vi "labview_nanonisKernel.vi"(3 "Error in (no error)":errorcluster, 4 "Input":string, 5 "Application ref in":refnum<vi>) -> (0 "Error out":errorcluster, 2 "Output":string)   [LabVIEW 2019]
uses:
  <userlib>/Nanonis Prog Interface/Scan/Grid/GridPatternGet.vi
  <userlib>/Nanonis Prog Interface/Nanonis Prog Interface.lvlib
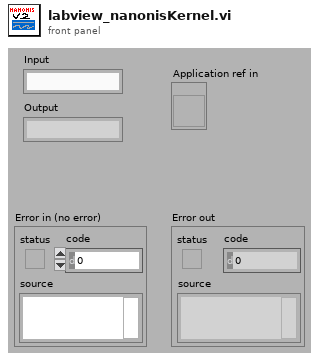
[diagram p1: front panel]
types:
  T1 = enum16{"no change", "home absolute", "home relative"}
  T2 = enum8{"Group 1", "Group 2", "Group 3", "Group 4", "Group 5", "Group 6"}
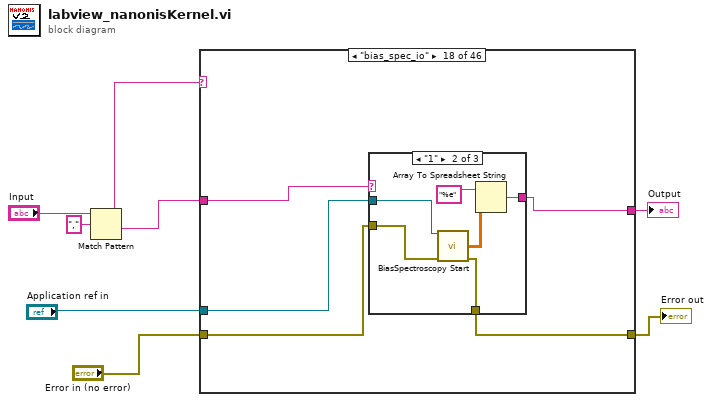
[diagram p0: block diagram]
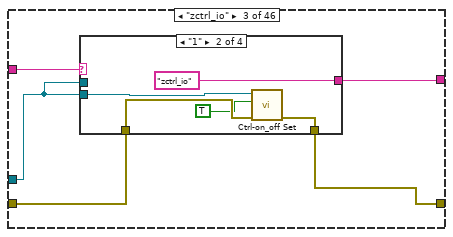
[diagram p4: hidden frame]
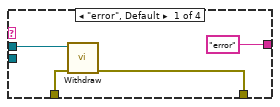
[diagram p5: hidden frame]
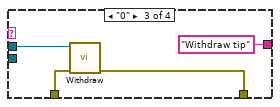
[diagram p6: hidden frame]
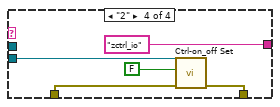
[diagram p7: hidden frame]
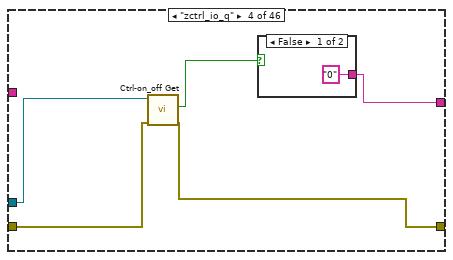
[diagram p8: hidden frame]
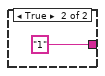
[diagram p9: hidden frame]
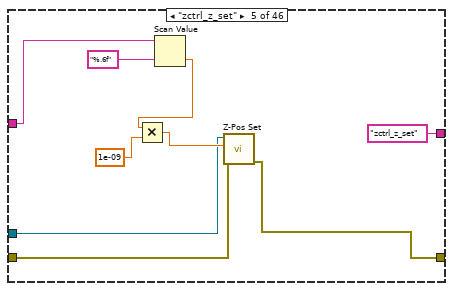
[diagram p10: hidden frame]
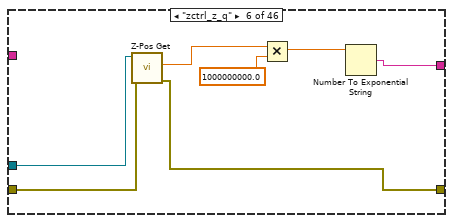
[diagram p11: hidden frame]
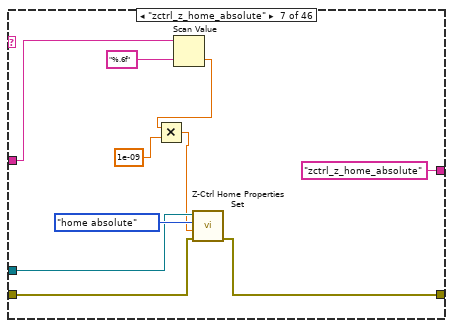
[diagram p12: hidden frame]
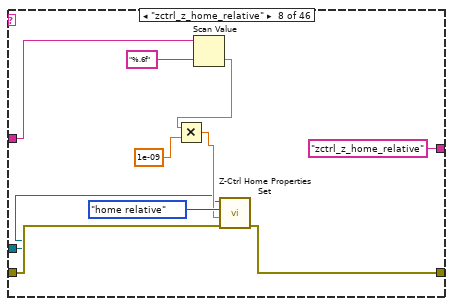
[diagram p13: hidden frame]
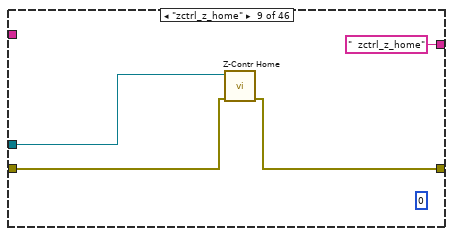
[diagram p14: hidden frame]
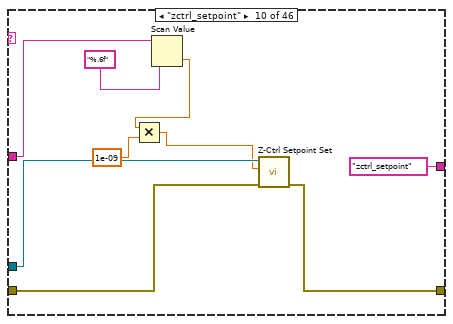
[diagram p15: hidden frame]
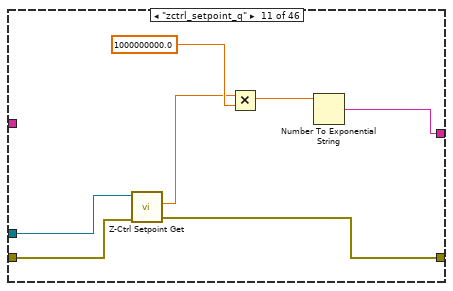
[diagram p16: hidden frame]
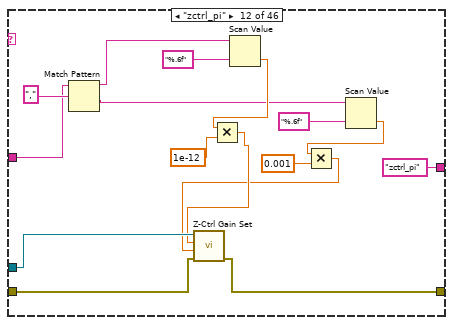
[diagram p17: hidden frame]
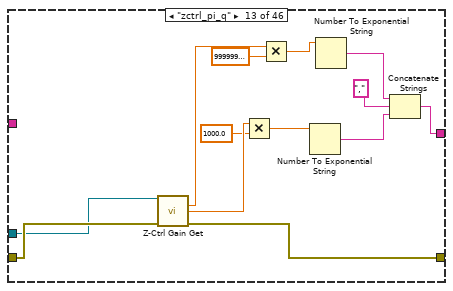
[diagram p18: hidden frame]
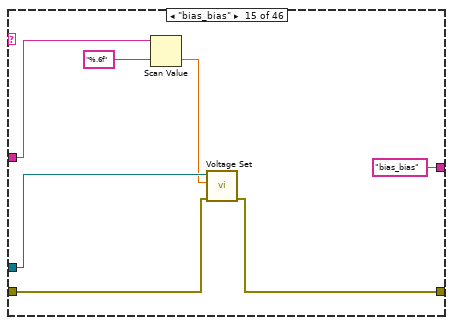
[diagram p20: hidden frame]
diagram:
  n1 = Match Pattern(string="Input", regular expression=",") -> (before substring=w5:string, after substring=w4:string)  [unwired: 1 in, 2 out]
  n2 = case shown="\"bias_spec_io\"" w5 {
    tunnel: [w10 w12 w16 w37 "zctrl_z_set" ("Input") w53 "zctrl_z_home_absolute" ("Input") "zctrl_z_home_relative" ("Input") "  zctrl_z_home" ("Input") "zctrl_setpoint" ("Input") w96 "zctrl_pi" ("Input") w115 w129 "bias_bias" ("Input") w138 "bias_pulse" ("Input") w163 w180 "bias_spec_sweep" ("Input") w199 "  bias_spec_channel" ("Input") w217 w219 w220 w223 w225 w227 w230 w255 w269 w295 w319 w330 w351 w360 w377 w389 w397 w412 w420 w436 "1" ("regular expression") w447 w461 w469] -> w8
    tunnel: w4 -> [w10 w12 w17 _ w50 _ w59 w69 _ w83 _ w106 _ w129 w130 _ w149 w162 _ w187 _ w213 w217 w219 w220 w223 w225 w227 w236 w256 w270 w297 w311 w342 w359 w365 w378 _ w408 _ _ w435 _ _ _ w469]
    tunnel: "Error in (no error)" -> [w9 w11 w15 w39 w45 w57 w66 w76 w82 w91 w94 w113 w127 w128 w136 w141 w156 w165 w178 w195 w204 w212 w216 w218 w221 w222 w224 w226 w235 w259 w272 w305 w326 w341 w355 w363 w376 w388 _ w418 w423 w432 w445 w451 w467 w478]
    tunnel: "Application ref in" -> [_ _ w14 w40 w46 w58 w64 w70 w79 w90 w95 w112 w125 _ w133 w140 w155 w161 w177 w193 w196 w210 _ _ _ _ _ _ w234 w260 w271 w306 w327 w340 w356 w364 w375 w386 w400 w419 w424 w431 w443 w450 w468 w476]
    tunnel: [w9 w11 w13 w36 w43 w52 w65 w75 w81 w89 w93 w111 w126 w128 w135 w139 w154 w164 w179 w194 w203 w211 w216 w218 w221 w222 w224 w226 w233 w246 w268 w302 w325 w335 w354 w361 w372 w387 w399 w417 w421 w430 w444 w449 w466 w477] -> w2
    frame "test", Default {
    }
    frame "###z controller###" {
    }
    frame "zctrl_io" {
      n3 = case shown="\"1\"" w17 {
        tunnel: ["error" ("regular expression") "zctrl_io" ("regular expression") "Withdraw tip" ("regular expression") "zctrl_io" ("regular expression")] -> w16
        tunnel: w14 -> [w19 _ w30 _]
        tunnel: w15 -> [w20 w25 w29 w31]
        tunnel: w14 -> [_ w23 _ w33]
        tunnel: [w18 w22 w27 w34] -> w13
        frame "error", Default {
          n4 = call <userlib>:"Withdraw.vi"("Error in (no error)"=w20, "Application ref in"=w19) -> ("Error out"=w18:errorcluster)  [unwired: 8 in, 1 out]
        }
        frame "1" {
          n5 = call <userlib>:"Ctrl-on_off Set.vi"("error in (no error)"=w25, "Z Controller ON/OFF"=TRUE ("Lockin ON/OFF"), "Application ref in"=w23) -> ("error out"=w22:errorcluster)  [unwired: 7 in, 1 out]
        }
        frame "0" {
          n6 = call <userlib>:"Withdraw.vi"("Error in (no error)"=w29, "Application ref in"=w30) -> ("Error out"=w27:errorcluster)  [unwired: 8 in, 1 out]
        }
        frame "2" {
          n7 = call <userlib>:"Ctrl-on_off Set.vi"("error in (no error)"=w31, "Z Controller ON/OFF"=FALSE ("Lockin ON/OFF"), "Application ref in"=w33) -> ("error out"=w34:errorcluster)  [unwired: 7 in, 1 out]
        }
      }
    }
    frame "zctrl_io_q" {
      n8 = call <userlib>:"Ctrl-on_off Get.vi"("error in (no error)"=w39, "Application ref in"=w40) -> ("error out"=w36:errorcluster, "Z-Controller on/off status"=w38:bool)  [unwired: 7 in, 1 out]
      n9 = case shown="False" w38 {
        tunnel: ["0" "1"] -> w37
        frame False {
        }
        frame True {
        }
      }
    }
    frame "zctrl_z_set" {
      n10 = Scan Value(string=w50, format string="%.6f") -> (value=w48:dbl)  [unwired: 1 in, 1 out]
      n11 = Multiply(x=w48, y=1e-09) -> (x*y=w47:dbl)
      n12 = call <userlib>:"Z-Pos Set.vi"("error in (no error)"=w45, "Z position (m)"=w47, "Application ref in"=w46) -> ("error out"=w43:errorcluster)  [unwired: 7 in, 1 out]
    }
    frame "zctrl_z_q" {
      n13 = call <userlib>:"Z-Pos Get.vi"("error in (no error)"=w57, "Application ref in"=w58) -> ("error out"=w52:errorcluster, "Z position (m)"=w55:sgl)  [unwired: 7 in, 1 out]
      n14 = Multiply(x=w55, y=1000000000.0) -> (x*y=w54:dbl)
      n15 = Number To Exponential String(number=w54) -> (E-format string=w53:string)  [unwired: 3 in]
    }
    frame "zctrl_z_home_absolute" {
      n16 = Scan Value(string=w59, format string="%.6f") -> (value=w61:dbl)  [unwired: 1 in, 1 out]
      n17 = Multiply(x=w61, y=1e-09) -> (x*y=w60:dbl)
      n18 = call <userlib>:"Z-Ctrl Home Properties Set.vi"("error in (no error)"=w66, "Home position (m) (NaN=no change)"=w60, "Absolute/Relative Switch (no change=Default)"=T1."home absolute", "Application ref in"=w64) -> ("error out"=w65:errorcluster)  [unwired: 5 in, 1 out]
    }
    frame "zctrl_z_home_relative" {
      n19 = Scan Value(string=w69, format string="%.6f") -> (value=w72:dbl)  [unwired: 1 in, 1 out]
      n20 = Multiply(x=w72, y=1e-09) -> (x*y=w71:dbl)
      n21 = call <userlib>:"Z-Ctrl Home Properties Set.vi"("error in (no error)"=w76, "Home position (m) (NaN=no change)"=w71, "Absolute/Relative Switch (no change=Default)"=T1."home relative", "Application ref in"=w70) -> ("error out"=w75:errorcluster)  [unwired: 5 in, 1 out]
    }
    frame "zctrl_z_home" {
      (unwired) 0
      n22 = call <userlib>:"Z-Contr Home.vi"("Error in (no error)"=w82, "Application ref in"=w79) -> ("Error out"=w81:errorcluster)  [unwired: 8 in, 1 out]
    }
    frame "zctrl_setpoint" {
      n23 = Scan Value(string=w83, format string="%.6f") -> (value=w86:dbl)  [unwired: 1 in, 1 out]
      n24 = Multiply(x=w86, y=1e-09) -> (x*y=w85:dbl)
      n25 = call <userlib>:"Z-Ctrl Setpoint Set.vi"("error in (no error)"=w91, "Z Controller setpoint"=w85, "Application ref in"=w90) -> ("error out"=w89:errorcluster)  [unwired: 7 in, 1 out]
    }
    frame "zctrl_setpoint_q" {
      n26 = call <userlib>:"Z-Ctrl Setpoint Get.vi"("error in (no error)"=w94, "Application ref in"=w95) -> ("error out"=w93:errorcluster, "Z Controller setpoint"=w92:sgl)  [unwired: 6 in, 1 out]
      n27 = Multiply(x=w92, y=1000000000.0) -> (x*y=w97:dbl)
      n28 = Number To Exponential String(number=w97) -> (E-format string=w96:string)  [unwired: 3 in]
    }
    frame "zctrl_pi" {
      n29 = Match Pattern(string=w106, regular expression=",") -> (before substring=w105:string, after substring=w102:string)  [unwired: 1 in, 2 out]
      n30 = Scan Value(string=w105, format string="%.6f") -> (value=w108:dbl)  [unwired: 1 in, 1 out]
      n31 = Multiply(x=w108, y=1e-12) -> (x*y=w104:dbl)
      n32 = Scan Value(string=w102, format string="%.6f") -> (value=w101:dbl)  [unwired: 1 in, 1 out]
      n33 = Multiply(x=w101, y=0.001) -> (x*y=w100:dbl)
      n34 = call <userlib>:"Z-Ctrl Gain Set.vi"("error in (no error)"=w113, "Time constant (s)"=w100, "P-gain"=w104, "Application ref in"=w112) -> ("error out"=w111:errorcluster)  [unwired: 5 in, 1 out]
    }
    frame "zctrl_pi_q" {
      n35 = call <userlib>:"Z-Ctrl Gain Get.vi"("Application ref in"=w125, "error in (no error)"=w127) -> ("P-gain"=w122:sgl, "Time constant (s)"=w121:sgl, "error out"=w126:errorcluster)  [unwired: 9 in, 2 out]
      n36 = Multiply(x=w121, y=sgl 1000.0) -> (x*y=w123:sgl)
      n37 = Multiply(x=w122, y=sgl 1000000000000.0) -> (x*y=w124:sgl)
      n38 = Number To Exponential String(number=w123) -> (E-format string=w116:string)  [unwired: 3 in]
      n39 = Number To Exponential String(number=w124) -> (E-format string=w117:string)  [unwired: 3 in]
      n40 = Concatenate Strings(w117, "," ("string"), w116) -> (w115:string)
    }
    frame "###Bias/Bias Spectrum###" {
    }
    frame "bias_bias" {
      n41 = Scan Value(string=w130, format string="%.6f") -> (value=w132:dbl)  [unwired: 1 in, 1 out]
      n42 = call <userlib>:"Voltage Set.vi"("Error in (no error)"=w136, "Bias (V)"=w132, "Application ref in"=w133) -> ("Error out"=w135:errorcluster)  [unwired: 7 in, 1 out]
    }
    frame "bias_bias_q" {
      n43 = call <userlib>:"Voltage Get.vi"("error in (no error)"=w141, "Application ref in"=w140) -> ("error out"=w139:errorcluster, "Bias (V)"=w137:sgl)  [unwired: 7 in, 1 out]
      n44 = Number To Exponential String(number=w137) -> (E-format string=w138:string)  [unwired: 3 in]
    }
    frame "bias_pulse" {
      w146 = "," ("regular expression")
      n45 = Match Pattern(string=w149, regular expression=w146) -> (before substring=w151:string, after substring=w144:string)  [unwired: 1 in, 2 out]
      n46 = Match Pattern(string=w144, regular expression=w146) -> (before substring=w145:string, after substring=w143:string)  [unwired: 1 in, 2 out]
      n47 = Scan Value(string=w151, format string="%.6f") -> (value=w148:dbl)  [unwired: 1 in, 1 out]
      n48 = case shown="\"0\"" w143 {
        tunnel: [enum16{"no change", "hold", "don't hold"}."no change" ("Z-Controller (no change)") enum16{"no change", "hold", "don't hold"}."hold" ("Z-Controller (no change)") enum16{"no change", "hold", "don't hold"}."don't hold" ("Z-Controller (no change)")] -> w142
        frame Default {
        }
        frame "1" {
        }
        frame "0" {
        }
      }
      n49 = Scan Value(string=w145, format string="%.6f") -> (value=w147:dbl)  [unwired: 1 in, 1 out]
      n50 = call <userlib>:"Bias Pulse.vi"("Application ref in"=w155, "Pulse bias (V) (1)"=w148, "Pulse width (s) (100m)"=w147, "Z-Controller (no change)"=w142, "Error in (no error)"=w156, "Pulse abs/rel (no change)"=enum16{"no change", "relative", "absolute"}."absolute") -> ("Error out"=w154:errorcluster)  [unwired: 8 in, 1 out]
    }
    frame "bias_spec_io" {
      n51 = case shown="\"1\"" w162 {
        tunnel: ["Error!" ("regular expression") w169 "STS stop" ("regular expression")] -> w163
        tunnel: w165 -> [w166 w172 w175]
        tunnel: w161 -> [_ w173 _]
        tunnel: [w166 w171 w174] -> w164
        frame "error", Default {
        }
        frame "1" {
          n52 = call <userlib>:"BiasSpectroscopy Start.vi"("Application ref in"=w173, "Error in (no error)"=w172) -> ("Data"=w168:sgl[][], "Error out"=w171:errorcluster)  [unwired: 9 in, 3 out]
          n53 = Array To Spreadsheet String(array=w168, 3:"%e" ("format string")) -> (spreadsheet string=w169:string)  [unwired: 1 in]
        }
        frame "0" {
          n54 = call <userlib>:"BiasSpectroscopy Stop.vi"("Error in (no error)"=w175) -> ("Error out"=w174:errorcluster)  [unwired: 13 in, 1 out]
        }
      }
    }
    frame "bias_spec_q" {
      n55 = call <userlib>:"BiasSpectroscopy Status Get.vi"("Error in (no error)"=w178, "Application ref in"=w177) -> ("Error out"=w179:errorcluster, "Running?"=w181:bool)  [unwired: 5 in, 1 out]
      n56 = case shown="True" w181 {
        tunnel: ["0" "1"] -> w180
        frame False {
        }
        frame True {
        }
      }
    }
    frame "bias_spec_sweep" {
      n57 = Match Pattern(string=w187, regular expression=",") -> (before substring=w190:string, after substring=w188:string)  [unwired: 1 in, 2 out]
      n58 = Scan Value(string=w190, format string="%.6f") -> (value=w186:dbl)  [unwired: 1 in, 1 out]
      n59 = Scan Value(string=w188, format string="%.6f") -> (value=w185:dbl)  [unwired: 1 in, 1 out]
      n60 = call <userlib>:"BiasSpectroscopy SetLimits.vi"("Error in (no error)"=w195, "End value (V)"=w185, "Start value (V)"=w186, "Application ref in"=w193) -> ("Error out"=w194:errorcluster)  [unwired: 4 in, 1 out]
    }
    frame "bias_spec_sweep_q" {
      n61 = call <userlib>:"BiasSpectroscopy GetLimits.vi"("Error in (no error)"=w204, "Application ref in"=w196) -> ("Error out"=w203:errorcluster, "End value (V)"=w198:sgl, "Start value (V)"=w197:sgl)  [unwired: 4 in, 1 out]
      n62 = Number To Exponential String(number=w198) -> (E-format string=w200:string)  [unwired: 3 in]
      n63 = Number To Exponential String(number=w197) -> (E-format string=w201:string)  [unwired: 3 in]
      n64 = Concatenate Strings(w201, "," ("string"), w200) -> (w199:string)
    }
    frame "bias_spec_channel" {
      n65 = Spreadsheet String To Array(delimiter (Tab)=",", format string="", spreadsheet string=w213) -> (array=w208:dbl[][])  [unwired: 1 in]
      n66 = Array Size(array=w208) -> (size(s)=w209:i32[])
      n67 = Array Max & Min(array=w209) -> (max value=w207:i32)  [unwired: 3 out]
      n68 = Reshape Array(w208, w207) -> (w206:dbl[])
      n69 = call <userlib>:"BiasSpectroscopy Channels Set.vi"("Error in (no error)"=w212, "Channels"=w206, "Application ref in"=w210) -> ("Error out"=w211:errorcluster)  [unwired: 7 in, 1 out]
    }
    frame "###Current###" {
    }
    frame "###Walker###" {
    }
    frame "###Move/Drift/Tilt###" {
    }
    frame "###Scan###" {
    }
    frame "###Grid###" {
    }
    frame "###LockIn###" {
    }
    frame "WLK_S" {
      w239 = "," ("regular expression")
      # "Frequency"
      # "Voltage"
      n70 = Match Pattern(string=w236, regular expression=w239) -> (before substring=w232:string, after substring=w240:string)  [unwired: 1 in, 2 out]
      n71 = Match Pattern(string=w240, regular expression=w239) -> (before substring=w231:string)  [unwired: 1 in, 3 out]
      n72 = Decimal String To Number(string=w231) -> (number=w238:i32)  [unwired: 2 in, 1 out]
      n73 = Decimal String To Number(string=w232) -> (number=w237:i32)  [unwired: 2 in, 1 out]
      n74 = call <userlib>:"Motor Frequency Amplitude Set.vi"("Error in (no error)"=w235, "Amplitude (V) (NaN=no change)"=w237, "Frequency (Hz) (NaN=no change)"=w238, "Application ref in"=w234) -> ("Error out"=w233:errorcluster)  [unwired: 6 in, 1 out]
      n75 = Concatenate Strings("WLK_S, V:  " ("string"), w232, ", F: " ("string"), w231) -> (w230:string)
    }
    frame "WLK_W" {
      w252 = "," ("string")
      # "Steps"
      # "Direction"
      n76 = Match Pattern(string=w256, regular expression=w252) -> (before substring=w242:string, after substring=w258:string)  [unwired: 1 in, 2 out]
      n77 = case shown="\"False\", Default" w242 {
        tunnel: [-1 0 1 2 3 4 5] -> w241
        frame "False", Default {
        }
        frame "+X", "+x", "0", "X+", "x+" {
        }
        frame "-X", "-x", "1", "X-", "x-" {
        }
        frame "+Y", "+y", "2", "Y+", "y+" {
        }
        frame "-Y", "-y", "3", "Y-", "y-" {
        }
        frame "+Z", "+z", "4", "Z+", "z+" {
        }
        frame "-Z", "-z", "5", "Z-", "z-" {
        }
      }
      n78 = Match Pattern(string=w258, regular expression=w252) -> (before substring=w257:string)  [unwired: 1 in, 3 out]
      n79 = Decimal String To Number(string=w257) -> (number=w250:i32)  [unwired: 2 in, 1 out]
      n80 = call <userlib>:"Motor Start Move.vi"("Group"=T2."Group 4", "Error in (no error)"=w259, "Number of steps"=w250, "Direction"=w241, "Application ref in"=w260) -> ("Error out"=w245:errorcluster, "Application ref out"=w251:refnum<vi>)  [unwired: 4 in]
      n81 = Concatenate Strings("WLK_W, Dir: " ("string"), w242, ", Steps: " ("string"), w257) -> (w255:string)
      n82 = call <userlib>:"Motor Frequency Amplitude Get.vi"("Application ref in"=w251) -> ("Frequency (Hz)"=w249:sgl)  [unwired: 7 in, 3 out]
      n83 = Divide(x=w250, y=w249) -> (x/y=w248:sgl)
      n84 = Add(x=w248, y=sgl 0.5) -> (x+y=w244:sgl)
      n85 = call "Time Delay"("error in (no error)"=w245, "Delay Time (s)"=w244) -> ("error out"=w246:errorcluster)  [unwired: 9 in]
    }
    frame "WLK_W5" {
      w281 = "," ("string")
      # "Steps"
      # "Direction"
      n86 = Match Pattern(string=w270, regular expression=w281) -> (before substring=w286:string, after substring=w287:string)  [unwired: 1 in, 2 out]
      n87 = Match Pattern(string=w287, regular expression=w281) -> (before substring=w285:string)  [unwired: 1 in, 3 out]
      n88 = Decimal String To Number(string=w285) -> (number=w279:i32)  [unwired: 2 in, 1 out]
      n89 = Decimal String To Number(string=w286) -> (number=w284:i32)  [unwired: 2 in, 1 out]
      n90 = Concatenate Strings("WLK_W, Dir: " ("string"), w286, ", Steps: " ("string"), w285) -> (w269:string)
      n91 = call <userlib>:"Motor Start Move.vi"("Group"=T2."Group 5", "Error in (no error)"=w272, "Number of steps"=w279, "Direction"=w284, "Application ref in"=w271) -> ("Error out"=w275:errorcluster, "Application ref out"=w280:refnum<vi>)  [unwired: 4 in]
      n92 = call <userlib>:"Motor Frequency Amplitude Get.vi"("Application ref in"=w280) -> ("Frequency (Hz)"=w278:sgl)  [unwired: 7 in, 3 out]
      n93 = Divide(x=w279, y=w278) -> (x/y=w277:sgl)
      n94 = Add(x=w277, y=sgl 0.5) -> (x+y=w274:sgl)
      n95 = call "Time Delay2"("error in (no error)"=w275, "Delay Time (s)"=w274) -> ("error out"=w268:errorcluster)  [unwired: 9 in]
    }
    frame "RD_I" {
      w300 = "," ("regular expression")
      # "AVG#"
      # "Index"
      n96 = Match Pattern(string=w297, regular expression=w300) -> (before substring=w299:string, after substring=w301:string)  [unwired: 1 in, 2 out]
      n97 = Match Pattern(string=w301, regular expression=w300) -> (before substring=w298:string)  [unwired: 1 in, 3 out]
      n98 = call <userlib>:"Signal Names Get.vi"("error in (no error)"=w305, "Application ref in"=w306) -> ("error out"=w304:errorcluster, "Signals Names"=w294:string[], "Application ref out"=w303:refnum<vi>)  [unwired: 5 in]
      n99 = Decimal String To Number(string=w298) -> (number=w296:i32)  [unwired: 2 in, 1 out]
      n100 = Decimal String To Number(string=w299) -> (number=w293:i32)  [unwired: 2 in, 1 out]
      n101 = Index Array(array=w294, index=w293) -> (element=w291:string)
      n102 = call "Nanonis_read IO.vi"("error in (no error)"=w304, "Num Average"=w296, "Signal index (0-23)"=w293, "Application ref in"=w303) -> ("error out"=w302:errorcluster, "DC value"=w289:ext)
      n103 = Format Value(format string="%e", value (0)=w289) -> (output string=w290:string)  [unwired: 1 in]
      n104 = Concatenate Strings(w291, "," ("string"), w290) -> (w295:string)
    }
    frame "APP" {
      w307 = "," ("regular expression")
      # "100ms"
      n105 = Match Pattern(string=w311, regular expression=w307) -> (before substring=w317:string, after substring=w318:string)  [unwired: 1 in, 2 out]
      n106 = Match Pattern(string=w318, regular expression=w307) -> (before substring=w316:string, after substring=w308:string)  [unwired: 1 in, 2 out]
      n107 = Match Pattern(string=w308, regular expression=w307) -> (before substring=w309:string)  [unwired: 1 in, 3 out]
      n108 = Decimal String To Number(string=w309) -> (number=w310:i32)  [unwired: 2 in, 1 out]
      n109 = Decimal String To Number(string=w316) -> (number=w314:i32)  [unwired: 2 in, 1 out]
      n110 = Multiply(x=w314, y=1000) -> (x*y=w312:i32)
      n111 = Decimal String To Number(string=w317) -> (number=w315:i32)  [unwired: 2 in, 1 out]
      n112 = call "Nanonis_autoAPP.vi"("Application reference"=w327, "steps"=w315, "Number of pulses"=w310, "Wait for motor (ms)"=w312, "Error in (no error)"=w326) -> ("Surface reached"=w324:bool, "Total steps"=w320:u32, "error out"=w325:errorcluster)  [unwired: 1 in]
      n113 = case shown="False" w324 {
        tunnel: ["0" ("regular expression") "1" ("regular expression")] -> w323
        frame False {
        }
        frame True {
        }
      }
      n114 = Number To Decimal String(number=w320) -> (decimal integer string=w321:string)  [unwired: 1 in]
      n115 = Concatenate Strings(w323, "," ("string"), w321) -> (w319:string)
    }
    frame "LCK_S" {
      w336 = "%.6f" ("format string")
      w343 = "," ("string")
      w332 = "," ("string")
      # "Frequency"
      # "Phase"
      # "Amplitude"
      n116 = Match Pattern(string=w342, regular expression=w343) -> (before substring=w334:string, after substring=w344:string)  [unwired: 1 in, 2 out]
      n117 = Match Pattern(string=w344, regular expression=w343) -> (before substring=w333:string, after substring=w345:string)  [unwired: 1 in, 2 out]
      n118 = Match Pattern(string=w345, regular expression=w343) -> (before substring=w331:string)  [unwired: 1 in, 3 out]
      n119 = Scan Value(string=w331, format string=w336) -> (value=w337:dbl)  [unwired: 1 in, 1 out]
      n120 = Decimal String To Number(string=w334) -> (number=w339:i32)  [unwired: 2 in, 1 out]
      n121 = Scan Value(string=w333, format string=w336) -> (value=w338:dbl)  [unwired: 1 in, 1 out]
      n122 = call <userlib>:"Lockin Modulation param Set.vi"("Application ref in"=w340, "Amplitude (mod. signal unit) (NaN = no change)"=w338, "Frequency (Hz) (NaN = no change)"=w339, "Ref Phase (deg) (NaN = no change)"=w337, "Error in (no error)"=w341) -> ("Error out"=w335:errorcluster)  [unwired: 9 in, 1 out]
      n123 = Concatenate Strings(w334, w332, w333, w332, w331) -> (w330:string)
    }
    frame "LCK_M" {
      w358 = "," ("regular expression")
      # "Demod"
      # "Mod"
      n124 = Match Pattern(string=w359, regular expression=w358) -> (before substring=w349:string, after substring=w357:string)  [unwired: 1 in, 2 out]
      n125 = Match Pattern(string=w357, regular expression=w358) -> (before substring=w346:string)  [unwired: 1 in, 3 out]
      n126 = Decimal String To Number(string=w349) -> (number=w353:i32)  [unwired: 2 in, 1 out]
      n127 = Decimal String To Number(string=w346) -> (number=w352:i32)  [unwired: 2 in, 1 out]
      n128 = call <userlib>:"Lockin MoDem Signal Set.vi"("Error in (no error)"=w355, "Demod. index"=w352, "Mod. index"=w353, "Application ref in"=w356) -> ("Error out"=w354:errorcluster)  [unwired: 6 in, 1 out]
      n129 = Concatenate Strings("Mod: " ("string"), w349, "," ("string"), "Demod" ("string"), w346) -> (w351:string)
    }
    frame "LCK_IO" {
      n130 = case shown="\"0\"" w365 {
        tunnel: [FALSE ("Lockin ON/OFF") TRUE ("Lockin ON/OFF") FALSE ("Lockin ON/OFF")] -> w362
        tunnel: ["Error!" ("regular expression") "Lockin on" ("regular expression") "Lockin off" ("regular expression")] -> w360
        frame "error", Default {
        }
        frame "1" {
        }
        frame "0" {
        }
      }
      n131 = call <userlib>:"Lockin on_off Set.vi"("Error in (no error)"=w363, "Lockin ON/OFF"=w362, "Application ref in"=w364) -> ("Error out"=w361:errorcluster)  [unwired: 7 in, 1 out]
    }
    frame "SCAN_IO" {
      (unwired) 0
      n132 = case shown="\"start\"" w378 {
        tunnel: ["Error!" ("regular expression") "Scan start" ("regular expression") "Scan stop" ("regular expression")] -> w377
        tunnel: [enum16{"Start", "Stop", "Pause", "Resume"}."Pause" ("Scan action (Start)") enum16{"Start", "Stop", "Pause", "Resume"}."Start" ("Scan action (Start)") enum16{"Start", "Stop", "Pause", "Resume"}."Stop" ("Scan action (Start)")] -> w374
        frame "error", Default {
        }
        frame "start" {
        }
        frame "stop" {
          (unwired) FALSE ("Lockin ON/OFF")
        }
      }
      n133 = call <userlib>:"Scan Action.vi"("error in (no error)"=w376, "Direction: up/down (T=up)"=TRUE, "Scan action (Start)"=w374, "Application ref in"=w375) -> ("error out"=w372:errorcluster)  [unwired: 5 in, 1 out]
    }
    frame "SCAN_STAT" {
      (unwired) 0
      n134 = call <userlib>:"Scan Status Get.vi"("error in (no error)"=w388, "Application ref in"=w386) -> ("error out"=w387:errorcluster, "Scanning?"=w385:bool)  [unwired: 6 in, 1 out]
      n135 = case shown="False" w385 {
        tunnel: ["0" "1"] -> w389
        frame False {
        }
        frame True {
        }
      }
    }
    frame "SCAN_FRAME" {
      (unwired) 0
      w403 = "," ("regular expression")
      # "size"
      # "Y"
      # "X"
      n136 = Match Pattern(string=w408, regular expression=w403) -> (before substring=w396:string, after substring=w409:string)  [unwired: 1 in, 2 out]
      n137 = Match Pattern(string=w409, regular expression=w403) -> (before substring=w394:string, after substring=w404:string)  [unwired: 1 in, 2 out]
      n138 = Match Pattern(string=w404, regular expression=w403) -> (before substring=w392:string)  [unwired: 1 in, 3 out]
      n139 = Fract/Exp String To Number(string=w396) -> (number=w407:dbl)  [unwired: 3 in, 1 out]
      n140 = Fract/Exp String To Number(string=w394) -> (number=w406:dbl)  [unwired: 3 in, 1 out]
      n141 = Fract/Exp String To Number(string=w392) -> (number=w402:dbl)  [unwired: 3 in, 1 out]
      n142 = Bundle(w402, w402) -> (w401:cluster{dbl, dbl})  [unwired: 1 in]
      n143 = Bundle(w407, w406) -> (w405:cluster{dbl, dbl})  [unwired: 1 in]
      n144 = call <userlib>:"ScanFrame Set.vi"("Application ref in"=w400, "Center coordinates (m)"=w405, "Size (m)"=w401) -> ("error out"=w399:errorcluster)  [unwired: 11 in, 1 out]
      n145 = Concatenate Strings("Frame set: X= " ("string"), w396, ", Y= " ("string"), w394, ", size= " ("string"), w392) -> (w397:string)
    }
    frame "SCAN_location" {
      (unwired) 0
      n146 = call <userlib>:"ScanFrame Get.vi"("Application ref in"=w419, "error in (no error)"=w418) -> ("Center coordinates (m)"=w416:cluster{"Xc":sgl, "Yc":sgl}, "error out"=w417:errorcluster)  [unwired: 9 in, 3 out]
      n147 = Unbundle(w416) -> ("Xc"=w414:sgl, "Yc"=w413:sgl)
      n148 = Number To Exponential String(number=w414) -> (E-format string=w415:string)  [unwired: 3 in]
      n149 = Number To Exponential String(number=w413) -> (E-format string=w411:string)  [unwired: 3 in]
      n150 = Concatenate Strings(w415, "," ("string"), w411) -> (w412:string)
    }
    frame "SCAN_size" {
      n151 = call <userlib>:"ScanFrame Get.vi"("Application ref in"=w424, "error in (no error)"=w423) -> ("Size (m)"=w422:cluster{"Width":sgl, "Height":sgl}, "error out"=w421:errorcluster)  [unwired: 9 in, 3 out]
      n152 = Unbundle(w422) -> ("Width"=w428:sgl, "Height"=w427:sgl)
      n153 = Number To Exponential String(number=w428) -> (E-format string=w429:string)  [unwired: 3 in]
      n154 = Number To Exponential String(number=w427) -> (E-format string=w426:string)  [unwired: 3 in]
      n155 = Concatenate Strings(w429, "," ("string"), w426) -> (w420:string)
    }
    frame "FOLLOW" {
      (unwired) 0
      w441 = "," ("regular expression")
      # "Y"
      # "X"
      n156 = Match Pattern(string=w435, regular expression=w441) -> (before substring=w439:string, after substring=w442:string)  [unwired: 1 in, 2 out]
      n157 = Match Pattern(string=w442, regular expression=w441) -> (before substring=w437:string)  [unwired: 1 in, 3 out]
      n158 = Fract/Exp String To Number(string=w439) -> (number=w434:dbl)  [unwired: 3 in, 1 out]
      n159 = Fract/Exp String To Number(string=w437) -> (number=w433:dbl)  [unwired: 3 in, 1 out]
      n160 = call <userlib>:"XY-Pos Set.vi"("error in (no error)"=w432, "Y (m)"=w433, "X (m)"=w434, "Application ref in"=w431) -> ("error out"=w430:errorcluster)  [unwired: 4 in, 1 out]
      n161 = Concatenate Strings("Move tot: X= " ("string"), w439, ", Y= " ("string"), w437) -> (w436:string)
    }
    frame "GRD_IO" {
      (unwired) 1
      n162 = call <userlib>:"Start Grid Experiment.vi"("Application ref in"=w443, "error in (no error)"=w445) -> ("error out"=w444:errorcluster)  [unwired: 16 in, 1 out]
    }
    frame "GRD_STAT" {
      (unwired) 0
      n163 = call <userlib>:"Grid Experiment Status Get.vi"("error in (no error)"=w451, "Application ref in"=w450) -> ("error out"=w449:errorcluster, "Running?"=w448:bool)  [unwired: 7 in, 1 out]
      n164 = case shown="False" w448 {
        tunnel: ["0" "1"] -> w447
        frame False {
        }
        frame True {
        }
      }
    }
    frame "GRD_pattn" {
      w456 = "," ("string")
      (unwired) 0
      n165 = call-poly <userlib>:"Grid Pattern Get.vi"("Application ref in"=w468, "error in (no error)"=w467) -> ("Height (m)"=w457:sgl, "Width (m)"=w458:sgl, "Center Xc (m)"=w460:sgl, "Center Yc (m)"=w459:sgl, "Angle (°)"=w454:sgl, "error out"=w466:errorcluster)  [unwired: 9 in, 3 out]
      n166 = Number To Exponential String(number=w457) -> (E-format string=w462:string)  [unwired: 3 in]
      n167 = Number To Exponential String(number=w460) -> (E-format string=w465:string)  [unwired: 3 in]
      n168 = Number To Exponential String(number=w459) -> (E-format string=w464:string)  [unwired: 3 in]
      n169 = Number To Exponential String(number=w458) -> (E-format string=w463:string)  [unwired: 3 in]
      n170 = Number To Exponential String(number=w454) -> (E-format string=w455:string)  [unwired: 3 in]
      n171 = Concatenate Strings(w465, w456, w464, w456, w463, w456, w462, w456, w455) -> (w461:string)
    }
    frame "SWP_limit" {
      w474 = "," ("regular expression")
      (unwired) 0
      # "End"
      # "Start"
      n172 = Match Pattern(string=w469, regular expression=w474) -> (before substring=w473:string, after substring=w475:string)  [unwired: 1 in, 2 out]
      n173 = Match Pattern(string=w475, regular expression=w474) -> (before substring=w472:string)  [unwired: 1 in, 3 out]
      n174 = Fract/Exp String To Number(string=w473) -> (number=w471:dbl)  [unwired: 3 in, 1 out]
      n175 = Fract/Exp String To Number(string=w472) -> (number=w470:dbl)  [unwired: 3 in, 1 out]
      n176 = call <userlib>:"BiasSpectroscopy SetLimits.vi"("Error in (no error)"=w478, "End value (V)"=w470, "Start value (V)"=w471, "Application ref in"=w476) -> ("Error out"=w477:errorcluster)  [unwired: 4 in, 1 out]
    }
  }
  "Output" <- w8
  "Error out" <- w2
